vi "Fitting Configuration.vi"() -> (0 "Na intial guess":dbl[](array[numeric]), 1 "Force Guess?":bool, 2 "Na Fitting Results Save Path":string[](array[string]), 3 "Rb Fitting Results Save Path":string[](array[string]), 4 "Rb intial guess":dbl[](array[numeric]), 5 "Fitting Type":u16(ring) items=["2D Gaussian", "2D Quadrupole", "Double Gaussian", "Double Quadrupole", "Triple Gaussian", "Penta Gaussian"], 7 "Direct Summing Cluster":T1)   [LabVIEW 2015]
panel:
  in  "Direct summing cluster":T1
  in  "Rb Fitting results save path":string[](array[string])
  in  "Rb5":dbl[](array[numeric])
  in  "Rb4":dbl[](array[numeric])
  in  "Rb3":dbl[](array[numeric])
  in  "Rb2":dbl[](array[numeric])
  in  "Rb1":dbl[](array[numeric])
  in  "Force guess？":bool
  in  "Na Fitting results save path":string[](array[string])
  in  "Na5":dbl[](array[numeric])
  in  "Na4":dbl[](array[numeric])
  in  "Na3":dbl[](array[numeric])
  in  "Na2":dbl[](array[numeric])
  in  "Na1":dbl[](array[numeric])
  in  "Cancel":bool
  in  "OK":bool
  in  "Fitting type":u16(ring) items=["2D Gaussian", "2D Quadrupole", "Double Gaussian", "Double Quadrupole", "Triple Gaussian", "Penta Gaussian"]
  # "1st Component"
  # "2nd Component"
  # "3rd Component"
  # "peak"
  # "xc"
  # "yc"
  # "sigx"
  # "sigy"
  # "peak"
  # "xc"
  # "yc"
  # "sigx"
  # "sigy"
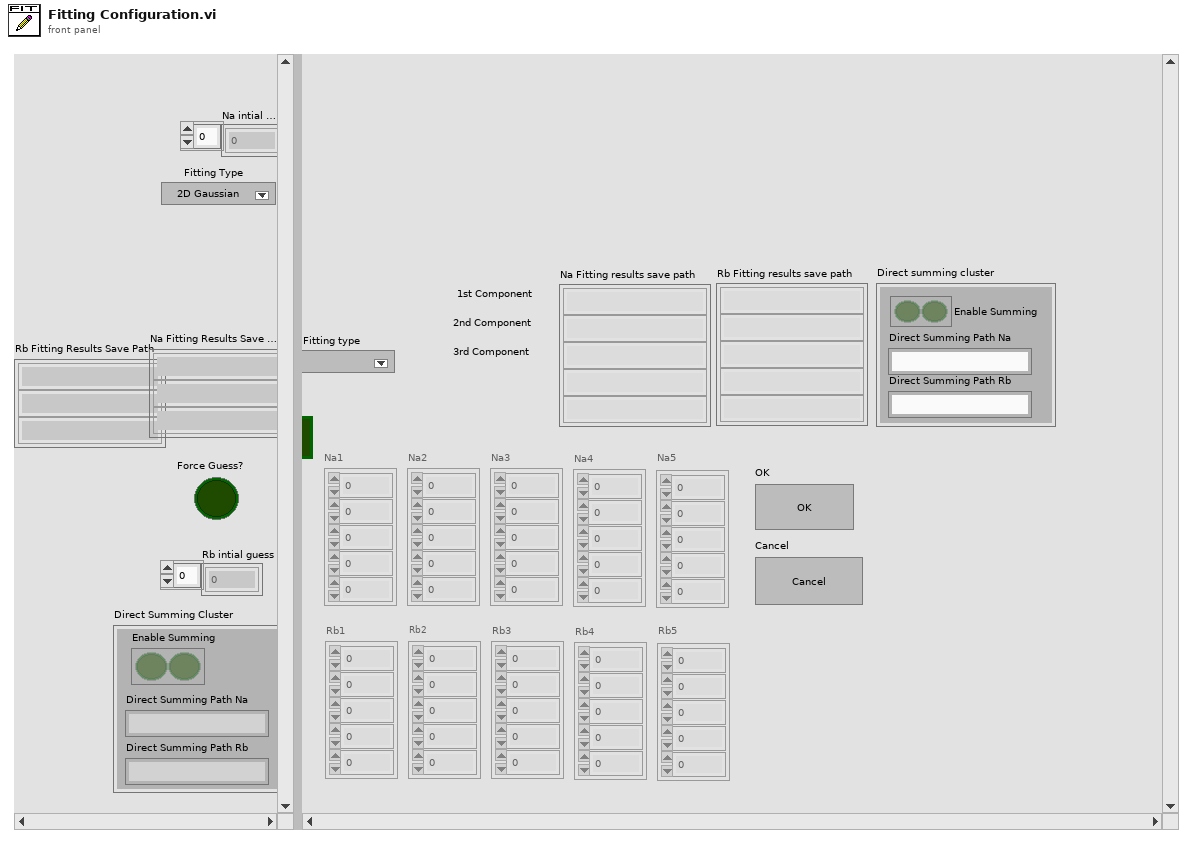
[diagram p1: front panel]
types:
  T1 = cluster{"Direct Summing Path Na":string, "Direct Summing Path Rb":string, "Enable Summing":bool[]}
  T2 = enum8{"Enabled", "Disabled", "Disabled and Grayed Out"}
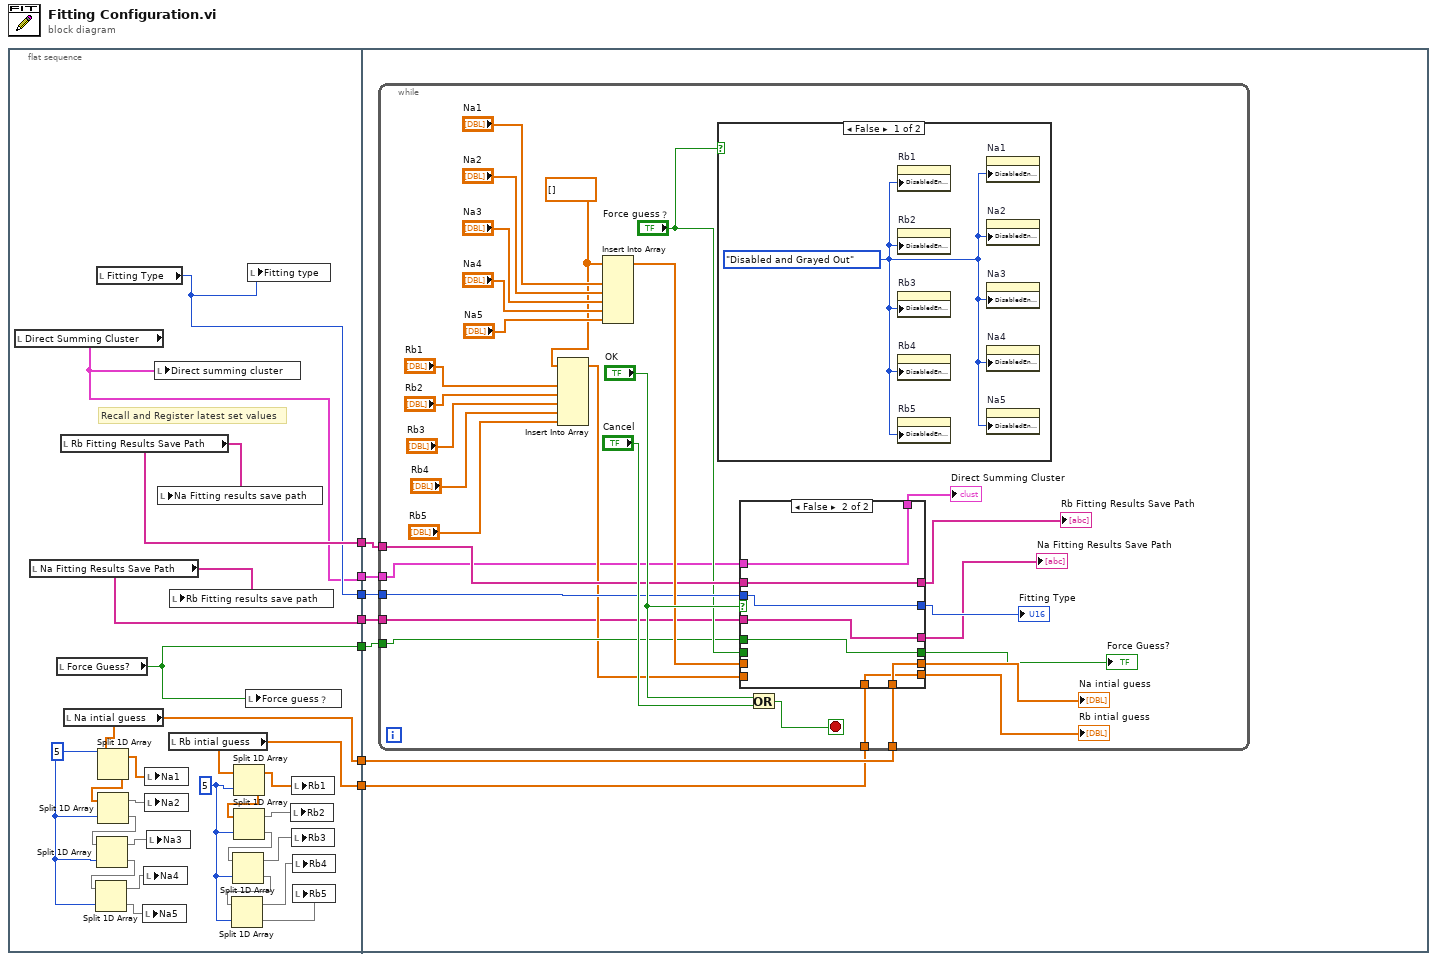
[diagram p0: block diagram]
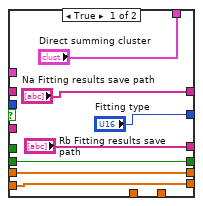
[diagram p2: hidden frame]
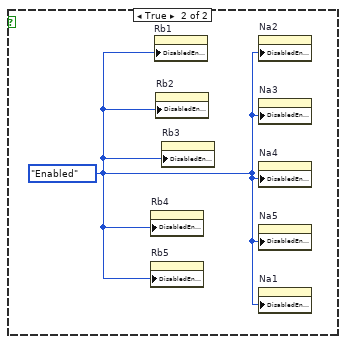
[diagram p3: hidden frame]
diagram:
  n1 = flat-sequence {
    tunnel: [w32] -> w7
    tunnel: [w31] -> w6
    tunnel: [w30] -> w5
    tunnel: [w29] -> w4
    tunnel: [w10] -> w3
    tunnel: [w9] -> w2
    tunnel: [w8] -> w1
    tunnel: w7 -> [w39]
    tunnel: w6 -> [w38]
    tunnel: w5 -> [w37]
    tunnel: w4 -> [w36]
    tunnel: w3 -> [w35]
    tunnel: w2 -> [w34]
    tunnel: w1 -> [w33]
    frame #0 {
      w18 = 5 ("index")
      w19 = 5 ("index")
      # "Recall and Register latest set values"
      n2 = local read "Direct Summing Cluster"() -> (w8:T1)
      n3 = local read "Na Fitting Results Save Path"() -> (w9:string[])
      n4 = local read "Force Guess?"() -> (w32:bool)
      n5 = local read "Rb Fitting Results Save Path"() -> (w31:string[])
      n6 = local read "Na intial guess"() -> (w29:dbl[])
      n7 = local read "Fitting Type"() -> (w30:u16)
      n8 = Split 1D Array(array=w29, index=w19) -> (first subarray=w28:dbl[], second subarray=w27:dbl[])
      n9 = Split 1D Array(array=w27, index=w19) -> (first subarray=w26:dbl[], second subarray=w25:dbl[])
      n10 = Split 1D Array(array=w25, index=w19) -> (first subarray=w24:dbl[], second subarray=w23:dbl[])
      n11 = Split 1D Array(array=w23, index=w19) -> (first subarray=w22:dbl[], second subarray=w21:dbl[])
      n12 = local write "Na5"(w21) -> ()
      n13 = local write "Na4"(w22) -> ()
      n14 = local write "Na1"(w28) -> ()
      n15 = local write "Na2"(w26) -> ()
      n16 = local write "Na3"(w24) -> ()
      n17 = local write "Direct summing cluster"(w8) -> ()
      n18 = local write "Na Fitting results save path"(w31) -> ()
      n19 = local read "Rb intial guess"() -> (w10:dbl[])
      n20 = local write "Rb Fitting results save path"(w9) -> ()
      n21 = Split 1D Array(array=w10, index=w18) -> (first subarray=w17:dbl[], second subarray=w20:dbl[])
      n22 = Split 1D Array(array=w20, index=w18) -> (first subarray=w16:dbl[], second subarray=w15:dbl[])
      n23 = Split 1D Array(array=w15, index=w18) -> (first subarray=w14:dbl[], second subarray=w13:dbl[])
      n24 = Split 1D Array(array=w13, index=w18) -> (first subarray=w12:dbl[], second subarray=w11:dbl[])
      n25 = local write "Force guess？"(w32) -> ()
      n26 = local write "Fitting type"(w30) -> ()
      n27 = local write "Rb2"(w16) -> ()
      n28 = local write "Rb1"(w17) -> ()
      n29 = local write "Rb3"(w14) -> ()
      n30 = local write "Rb4"(w12) -> ()
      n31 = local write "Rb5"(w11) -> ()
    }
    frame #1 {
      n32 = while {
        tunnel: w39 -> [w54]
        tunnel: w38 -> [w57]
        tunnel: w37 -> [w56]
        tunnel: w36 -> [w53]
        tunnel: w35 -> [w44]
        tunnel: w34 -> [w43]
        tunnel: w33 -> [w40]
        stop <- w70 stop-if-true
        w52 = dbl[] [] ("数组")
        n33 = Insert Into Array(array=w52, new element #1="Rb1", new element #2="Rb2", new element #3="Rb3", new element #4="Rb4", new element #5="Rb5") -> (w46:dbl[])  [unwired: 1 in]
        n34 = Insert Into Array(array=w52, new element #1="Na1", new element #2="Na2", new element #3="Na3", new element #4="Na4", new element #5="Na5") -> (w62:dbl[])  [unwired: 1 in]
        n35 = case shown="False" "Force guess？" {
          frame False {
            w85 = T2."Disabled and Grayed Out" ("禁用")
            n36 = property on="Rb1" class="Arr (strict)"("DisabledEnum"=w85) -> ()  [unwired: 2 in, 2 out]
            n37 = property on="Rb2" class="Arr (strict)"("DisabledEnum"=w85) -> ()  [unwired: 2 in, 2 out]
            n38 = property on="Rb3" class="Arr (strict)"("DisabledEnum"=w85) -> ()  [unwired: 2 in, 2 out]
            n39 = property on="Rb4" class="Arr (strict)"("DisabledEnum"=w85) -> ()  [unwired: 2 in, 2 out]
            n40 = property on="Rb5" class="Arr (strict)"("DisabledEnum"=w85) -> ()  [unwired: 2 in, 2 out]
            n41 = property on="Na1" class="Arr (strict)"("DisabledEnum"=w85) -> ()  [unwired: 2 in, 2 out]
            n42 = property on="Na2" class="Arr (strict)"("DisabledEnum"=w85) -> ()  [unwired: 2 in, 2 out]
            n43 = property on="Na3" class="Arr (strict)"("DisabledEnum"=w85) -> ()  [unwired: 2 in, 2 out]
            n44 = property on="Na4" class="Arr (strict)"("DisabledEnum"=w85) -> ()  [unwired: 2 in, 2 out]
            n45 = property on="Na5" class="Arr (strict)"("DisabledEnum"=w85) -> ()  [unwired: 2 in, 2 out]
          }
          frame True {
            w86 = T2."Enabled" ("禁用")
            n46 = property on="Rb4" class="Arr (strict)"("DisabledEnum"=w86) -> ()  [unwired: 2 in, 2 out]
            n47 = property on="Rb5" class="Arr (strict)"("DisabledEnum"=w86) -> ()  [unwired: 2 in, 2 out]
            n48 = property on="Rb1" class="Arr (strict)"("DisabledEnum"=w86) -> ()  [unwired: 2 in, 2 out]
            n49 = property on="Rb2" class="Arr (strict)"("DisabledEnum"=w86) -> ()  [unwired: 2 in, 2 out]
            n50 = property on="Rb3" class="Arr (strict)"("DisabledEnum"=w86) -> ()  [unwired: 2 in, 2 out]
            n51 = property on="Na2" class="Arr (strict)"("DisabledEnum"=w86) -> ()  [unwired: 2 in, 2 out]
            n52 = property on="Na3" class="Arr (strict)"("DisabledEnum"=w86) -> ()  [unwired: 2 in, 2 out]
            n53 = property on="Na4" class="Arr (strict)"("DisabledEnum"=w86) -> ()  [unwired: 2 in, 2 out]
            n54 = property on="Na5" class="Arr (strict)"("DisabledEnum"=w86) -> ()  [unwired: 2 in, 2 out]
            n55 = property on="Na1" class="Arr (strict)"("DisabledEnum"=w86) -> ()  [unwired: 2 in, 2 out]
          }
        }
        n56 = case shown="False" "OK" {
          tunnel: w62 -> [w77 _]
          tunnel: [w77 w81] -> w61
          tunnel: [w74 w82] -> w60
          tunnel: ["Fitting type" w83] -> w59
          tunnel: ["Na Fitting results save path" w84] -> w58
          tunnel: w57 -> [_ w84]
          tunnel: w56 -> [_ w83]
          tunnel: "Force guess？" -> [w74 _]
          tunnel: w54 -> [_ w82]
          tunnel: w53 -> [_ w81]
          tunnel: w46 -> [w73 _]
          tunnel: [w73 w80] -> w45
          tunnel: w44 -> [_ w80]
          tunnel: w43 -> [_ w79]
          tunnel: ["Rb Fitting results save path" w79] -> w42
          tunnel: ["Direct summing cluster" w78] -> w41
          tunnel: w40 -> [_ w78]
          frame True {
          }
          frame False {
          }
        }
        "Na intial guess" <- w61
        "Force Guess?" <- w60
        "Fitting Type" <- w59
        "Rb Fitting Results Save Path" <- w58
        "Rb intial guess" <- w45
        "Na Fitting Results Save Path" <- w42
        "Direct Summing Cluster" <- w41
        n57 = Or(x="OK", y="Cancel") -> (x .or. y?=w70:bool)
      }
    }
  }
